vi "PromptForAttributes.vi"(9 "Attributes In":string[][](array[string]), 10 "Mouse Coords":T1, 11 "New Node Name":string) -> (2 "Canceled":bool, 3 "Attributes":string[][](array[string]))   [LabVIEW 2017]
uses:
  <vilib>/Utility/miscctls.llb/LVPoint32TypeDef.ctl
  <vilib>/Utility/Data Type/NI_Data Type.lvlib
panel:
  out "Array":variant[](array[variant])
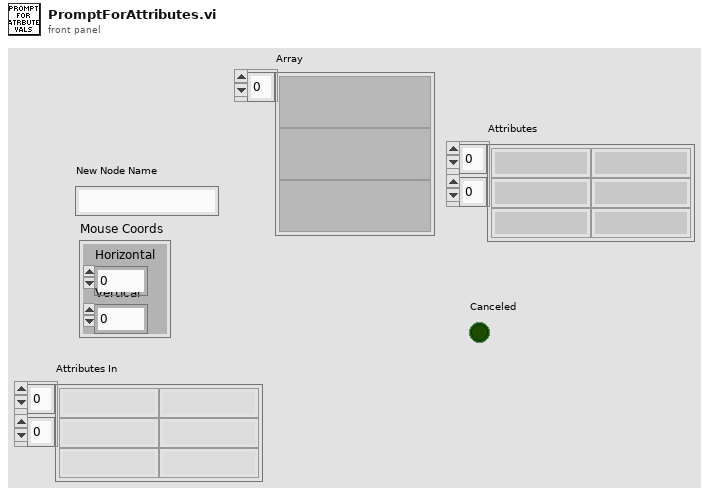
[diagram p1: front panel]
types:
  T1 = typedef "LVPoint32TypeDef.ctl" = cluster{"Horizontal":i32, "Vertical":i32}
  T2 = cluster{"Horizontal":i32, "Vertical":i32, "Horizontal":i32, "Vertical":i32}
  T3 = typedef "NI_Data Type.lvlib/Data Type.ctl" = enum8{"Invalid Type", "Void", "I8", "I16", "I32", "I64", "U8", "U16", "U32", "U64", "Single Float", "Double Float", "Extended Float", "Single Complex", "Double Complex", "Extended Complex", "Enum U8", "Enum U16", "Enum U32", "Enum U64", "Single Float With Unit", "Double Float With Unit", "Extended Float With Unit", "Single Complex with Unit", "Double Complex with Unit", "Extended Complex with Unit", "Boolean", "String", "Path", "Picture", "Tag", "Array", "Cluster", "Variant", "LV Variant", "Waveform", "Timestamp", "Digital Waveform", "Digital Data", "ExpressData", "Refnum", "External Data", "VI", "Poly VI", "LabVIEW Class Instance", "Fixed Point"}
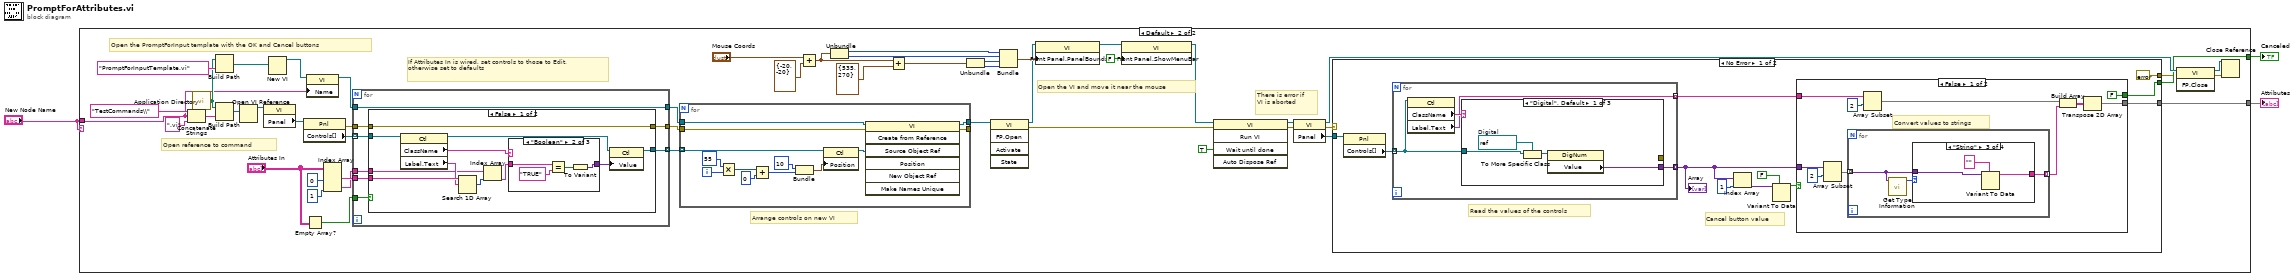
[diagram p0: block diagram]
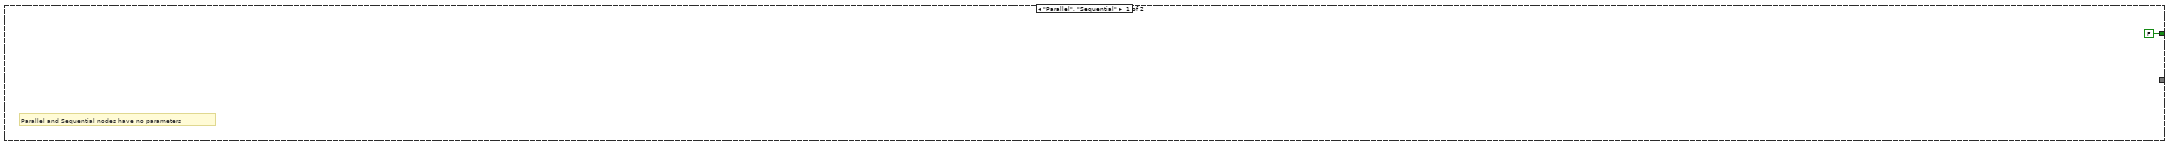
[diagram p2: hidden frame]
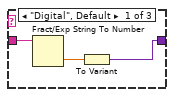
[diagram p3: hidden frame]
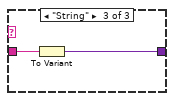
[diagram p4: hidden frame]
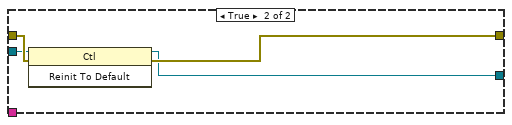
[diagram p5: hidden frame]
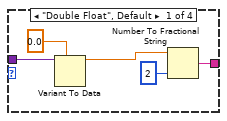
[diagram p6: hidden frame]
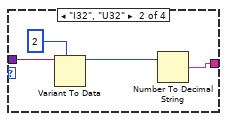
[diagram p7: hidden frame]
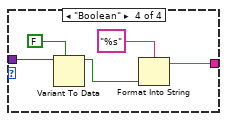
[diagram p8: hidden frame]
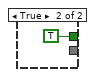
[diagram p9: hidden frame]
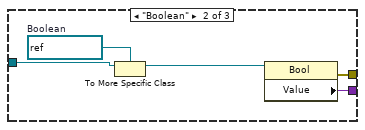
[diagram p10: hidden frame]
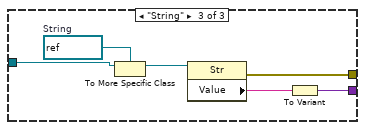
[diagram p11: hidden frame]
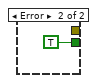
[diagram p12: hidden frame]
diagram:
  n1 = case shown="Default" "New Node Name" {
    tunnel: "New Node Name" -> [_ w5]
    tunnel: [FALSE ("Canceled") w38] -> w2
    tunnel: [_ w37] -> w1
    frame "Parallel", "Sequential" {
      # "Parallel and Sequential nodes have no parameters"
    }
    frame Default {
      # "There is error if\nVI is aborted"
      # "Open reference to command"
      # "Open the VI and move it near the mouse"
      # "Arrange controls on new VI"
      # "If Attributes In is wired, set controls to those to Edit,\notherwise set to defaults"
      # "Open the PromptForInput template with the OK and Cancel buttons"
      n2 = Concatenate Strings("TestCommands\\" ("string"), w5, ".vi" ("string")) -> (w42:string)
      n3 = call <vilib>:"Application Directory.vi"() -> ("Application Directory"=w41:path)
      n4 = Build Path(base path=w41, name or relative path="PromptForInputTemplate.vi") -> (appended path=w45:path)
      n5 = Build Path(base path=w41, name or relative path=w42) -> (appended path=w40:path)
      n6 = Open VI Reference(vi path=w40) -> (vi reference=w22:refnum<vi>)  [unwired: 5 in, 1 out]
      n7 = property class="VI"(reference=w22) -> ("Panel"=w54:refnum<vi>)  [unwired: 1 in, 2 out]
      n8 = New VI(10:w45) -> (3:w49:refnum<vi>)  [unwired: 6 in, 1 out]
      n9 = property class="Pnl"(reference=w54) -> (error out=w14:errorcluster, "Controls[]"=w17:refnum<vi>[])  [unwired: 1 in, 1 out]
      n10 = property class="VI"(reference=w49, "Name"=w5) -> (reference out=w12:refnum<vi>)  [unwired: 1 in, 1 out]
      n11 = Empty Array?(array="Attributes In") -> (empty?=w6:bool)
      n12 = Index Array(array="Attributes In", index (col) #1=0 ("disabled index (col)"), index (col) #2=1 ("index (col)")) -> (element #1=w10:string[], element #2=w8:string[])  [unwired: 2 in]
      n13 = for {
        tunnel: w17 -> [w60] mode=indexing
        tunnel: [w61] -> w16 mode=indexing
        tunnel: [w55] -> w15
        tunnel: w14 -> [w56]
        tunnel: [w62] -> w13
        tunnel: w12 -> [w62]
        tunnel: w10 -> [w59]
        tunnel: w8 -> [w58]
        tunnel: w6 -> [w57]
        n14 = case shown="False" w57 {
          tunnel: [w64 w84] -> w61
          tunnel: w60 -> [w73 w83]
          tunnel: w59 -> [w71 _]
          tunnel: w58 -> [w69 _]
          tunnel: w56 -> [w65 w86]
          tunnel: [w65 w85] -> w55
          frame False {
            n15 = property class="Ctl"(reference=w73) -> (reference out=w63:refnum<vi>, "ClassName"=w72:string, "Label.Text"=w70:string)  [unwired: 1 in, 1 out]
            n16 = Search 1D Array(1D array=w71, element=w70) -> (index of element=w68:i32)  [unwired: 1 in]
            n17 = Index Array(array=w69, index=w68) -> (element=w67:string)
            n18 = case shown="\"Boolean\"" w72 {
              tunnel: w67 -> [w76 w80 w82]
              tunnel: [w74 w77 w81] -> w66
              frame "Digital", Default {
                n19 = Fract/Exp String To Number(string=w76) -> (number=w75:dbl)  [unwired: 3 in, 1 out]
                n20 = To Variant(anything=w75) -> (Variant=w74:variant)
              }
              frame "Boolean" {
                n21 = Equal?(x=w80, y="TRUE") -> (x = y?=w78:bool)
                n22 = To Variant(anything=w78) -> (Variant=w77:variant)
              }
              frame "String" {
                n23 = To Variant(anything=w82) -> (Variant=w81:variant)
              }
            }
            n24 = property class="Ctl"(reference=w63, "Value"=w66) -> (reference out=w64:refnum<vi>)  [unwired: 1 in, 1 out]
          }
          frame True {
            n25 = invoke class="Ctl" method="Reinit To Default"(reference=w83, error in=w86) -> (reference out=w84:refnum<vi>, error out=w85:errorcluster)  [unwired: 1 in, 1 out]
          }
        }
      }
      n26 = for {
        tunnel: w13 -> [w161]
        tunnel: w15 -> [w160]
        tunnel: w16 -> [w149] mode=indexing
        tunnel: [w159] -> w18
        tunnel: [w158] -> _
        i -> [w157]
        n27 = Multiply(x=55, y=w157) -> (x*y=w155:i32)
        n28 = Add(x=w155, y=0) -> (x+y=w152:i32)
        n29 = Bundle("y"=10, w152) -> (w150:cluster{"y":i32, i32})  [unwired: 1 in]
        n30 = property class="Ctl"(reference=w149, "Position"=w150) -> (reference out=w153:refnum<vi>)  [unwired: 1 in, 1 out]
        n31 = invoke class="VI" method="Create from Reference"(reference=w161, error in=w160, "Source Object Ref"=w153) -> (reference out=w159:refnum<vi>, error out=w158:errorcluster)  [unwired: 4 in, 5 out]
      }
      n32 = Add(x="Mouse Coords", y=T1 {"Horizontal"=-20, "Vertical"=-20}) -> (x+y=w24:T1)
      n33 = Unbundle(w24) -> ("Horizontal"=w31:i32, "Vertical"=w30:i32)
      n34 = Add(x=w24, y=cluster{"Left":i16, "Top":i16} {"Left"=535, "Top"=270} ("Front Panel Window:Panel Bounds")) -> (x+y=w33:T1)
      n35 = Unbundle(w33) -> ("Horizontal"=w29:i32, "Vertical"=w28:i32)
      n36 = invoke class="VI" method="FP.Open"(reference=w18) -> (reference out=w21:refnum<vi>, error out=w48:errorcluster)  [unwired: 4 in, 3 out]
      n37 = Bundle("Horizontal"=w31, "Vertical"=w30, "Horizontal"=w29, "Vertical"=w28) -> (w27:T2)  [unwired: 1 in]
      n38 = property class="VI"(reference=w21, "Front Panel.PanelBounds"=w27) -> (reference out=w20:refnum<vi>)  [unwired: 1 in, 1 out]
      n39 = property class="VI"(reference=w20, "Front Panel.ShowMenuBar"=FALSE ("Front Panel Window:Show Menu Bar")) -> (reference out=w19:refnum<vi>)  [unwired: 1 in, 1 out]
      n40 = invoke class="VI" method="Run VI"(reference=w19, error in=w48, "Wait until done"=TRUE ("Wait Until Done")) -> (reference out=w50:refnum<vi>, error out=w51:errorcluster)  [unwired: 2 in, 3 out]
      n41 = property class="VI"(reference=w50, error in=w51) -> (reference out=w53:refnum<vi>, error out=w39:errorcluster, "Panel"=w52:refnum<vi>)
      n42 = case shown="No Error" w39 {
        tunnel: w52 -> [w96 _]
        tunnel: [w92 TRUE ("Canceled")] -> w38
        tunnel: [w89 _] -> w37
        tunnel: [errorcluster {"status"=FALSE, "code"=0, "source"=""} ("error constant") _] -> w34
        frame No Error {
          # "Cancel button value"
          # "Read the values of the controls"
          n43 = property class="Pnl"(reference=w96) -> ("Controls[]"=w97:refnum<vi>[])  [unwired: 1 in, 2 out]
          n44 = for {
            tunnel: w97 -> [w132] mode=indexing
            tunnel: [w130] -> w91 mode=indexing
            tunnel: [w129] -> w88 mode=indexing
            n45 = property class="Ctl"(reference=w132) -> ("ClassName"=w131:string, "Label.Text"=w129:string)  [unwired: 1 in, 2 out]
            n46 = case shown="\"Digital\", Default" w131 {
              tunnel: [_ w139 w145] -> _
              tunnel: w132 -> [w134 w138 w144]
              tunnel: [w133 w137 w142] -> w130
              frame "Digital", Default {
                w136 = refnum<vi> refnum  # Digital
                n47 = To More Specific Class(target class=w136, reference=w134) -> (specific class reference=w135:refnum<vi>)  [unwired: 1 in, 1 out]
                n48 = property class="DigNum"(reference=w135) -> ("Value"=w133:variant)  [unwired: 1 in, 2 out]
              }
              frame "Boolean" {
                w141 = refnum<vi> refnum  # Boolean
                n49 = To More Specific Class(target class=w141, reference=w138) -> (specific class reference=w140:refnum<vi>)  [unwired: 1 in, 1 out]
                n50 = property class="Bool"(reference=w140) -> (error out=w139:errorcluster, "Value"=w137:variant)  [unwired: 1 in, 1 out]
              }
              frame "String" {
                w147 = refnum<vi> refnum  # String
                n51 = To More Specific Class(target class=w147, reference=w144) -> (specific class reference=w146:refnum<vi>)  [unwired: 1 in, 1 out]
                n52 = property class="Str"(reference=w146) -> (error out=w145:errorcluster, "Value"=w143:string)  [unwired: 1 in, 1 out]
                n53 = To Variant(anything=w143) -> (Variant=w142:variant)
              }
            }
          }
          "Array" <- w91
          n54 = Index Array(array=w91, index=1) -> (element=w95:variant)
          n55 = Variant To Data(type=FALSE, Variant=w95) -> (data=w93:bool)  [unwired: 1 in, 1 out]
          n56 = case shown="False" w93 {
            tunnel: [FALSE ("Wait Until Done") TRUE ("Wait Until Done")] -> w92
            tunnel: w91 -> [w106 _]
            tunnel: [w98 _] -> w89
            tunnel: w88 -> [w101 _]
            frame False {
              # "Convert values to strings"
              n57 = Array Subset(array=w106, index=2) -> (w104:variant[])  [unwired: 1 in]
              n58 = for {
                tunnel: w104 -> [w109] mode=indexing
                tunnel: [w108] -> w103 mode=indexing
                n59 = call <vilib>:"Get Type Information.vi"("Variant"=w109) -> ("Type"=w110:T3)  [unwired: 6 in, 4 out]
                n60 = case shown="\"String\"" w110 {
                  tunnel: w109 -> [w113 w118 w122 w127]
                  tunnel: [w111 w117 w120 w125] -> w108
                  frame "Double Float", Default {
                    n61 = Variant To Data(type=0.0, Variant=w113) -> (data=w115:dbl)  [unwired: 1 in, 1 out]
                    n62 = Number To Fractional String(number=w115, precision (6)=i16 2) -> (F-format string=w111:string)  [unwired: 2 in]
                  }
                  frame "I32", "U32" {
                    n63 = Variant To Data(type=i16 2 ("precision (6)"), Variant=w118) -> (data=w119:i16)  [unwired: 1 in, 1 out]
                    n64 = Number To Decimal String(number=w119) -> (decimal integer string=w117:string)  [unwired: 1 in]
                  }
                  frame "String" {
                    n65 = Variant To Data(type="", Variant=w122) -> (data=w120:string)  [unwired: 1 in, 1 out]
                  }
                  frame "Boolean" {
                    n66 = Variant To Data(type=FALSE ("Wait Until Done"), Variant=w127) -> (data=w123:bool)  [unwired: 1 in, 1 out]
                    n67 = Format Into String(format string="%s", w123) -> (resulting string=w125:string)  [unwired: 2 in, 1 out]
                  }
                }
              }
              n68 = Array Subset(array=w101, index=2) -> (w100:string[])  [unwired: 1 in]
              n69 = Build Array(w100, w103) -> (w99:string[][])
              n70 = Transpose 2D Array(2D array=w99) -> (transposed array=w98:string[][])
            }
            frame True {
            }
          }
        }
        frame Error {
        }
      }
      n71 = invoke class="VI" method="FP.Close"(reference=w53, error in=w34) -> (reference out=w36:refnum<vi>, error out=w35:errorcluster)  [unwired: 1 in, 1 out]
      n72 = Close Reference(reference=w36, error in (no error)=w35) -> ()  [unwired: 1 out]
    }
  }
  "Attributes" <- w1
  "Canceled" <- w2
